vi "Launcher.vi"() -> ()   [LabVIEW 2014]
uses:
  Communication/Events/Events Lib.lvlib
  Communication/Queues/Queues Lib.lvlib
panel:
  in  "error in":errorcluster
  out "error out":errorcluster
  in  "Start Module":bool
  out "Log":string
  in  "Send Value to Chart":bool
  in  "Value":dbl
  in  "Stop Module":bool
  in  "Hide UI":bool
  in  "Show UI":bool
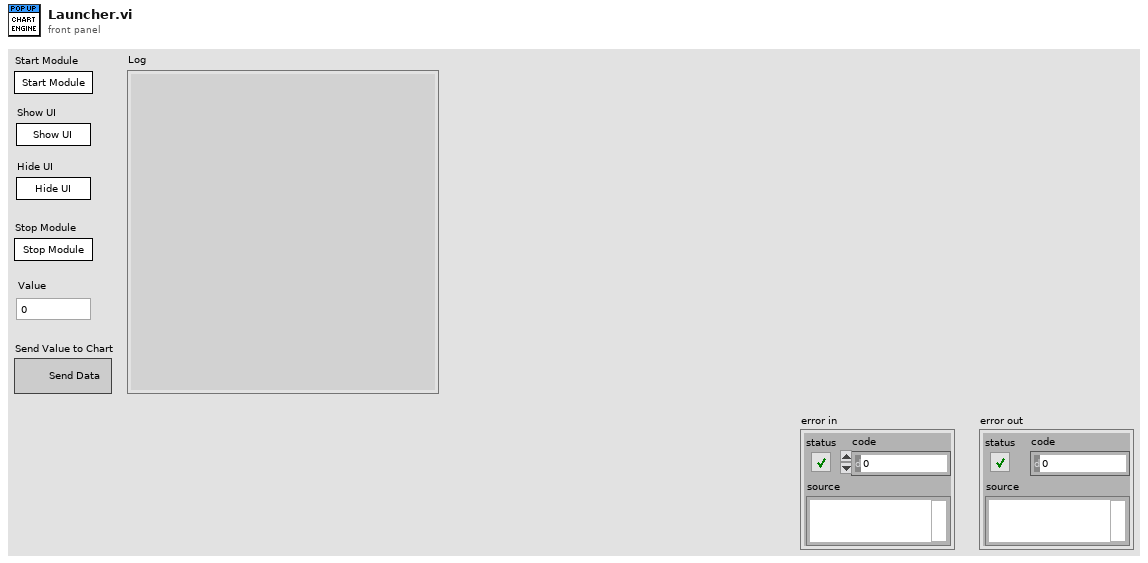
[diagram p1: front panel]
types:
  T1 = typedef "Events Lib.lvlib/Events TypeDef.ctl" = cluster{"Stop Event":refnum<user-event>, "Chart Send Value":refnum<user-event>, "Show Module":refnum<user-event>, "Hide Module":refnum<user-event>}
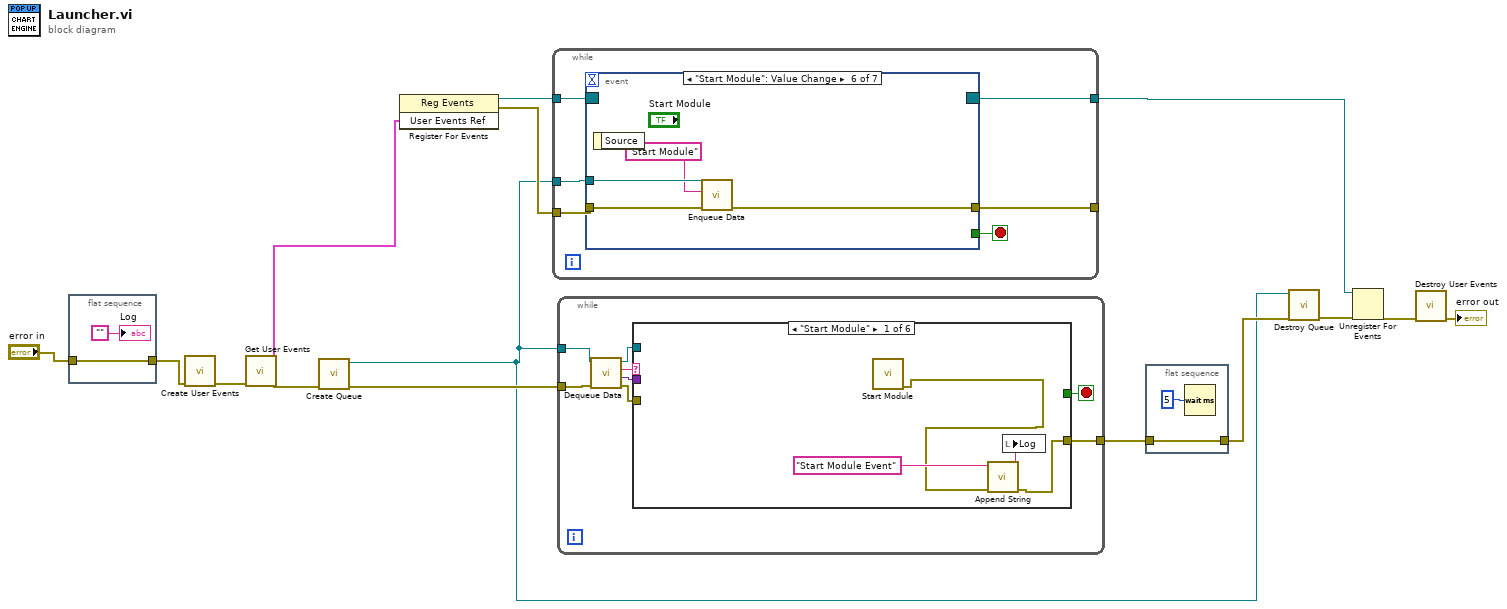
[diagram p0: block diagram]
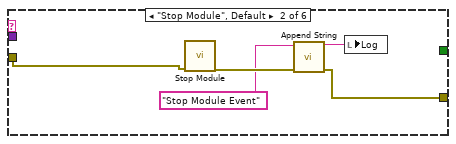
[diagram p2: hidden frame]
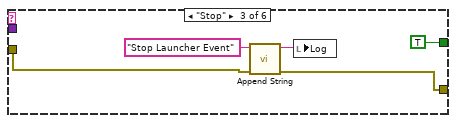
[diagram p3: hidden frame]
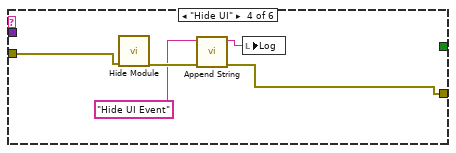
[diagram p4: hidden frame]
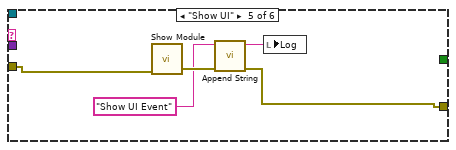
[diagram p5: hidden frame]
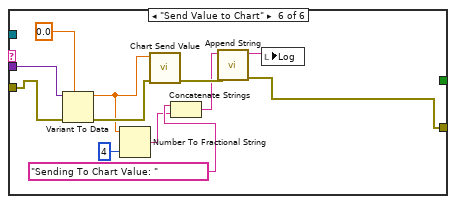
[diagram p6: hidden frame]
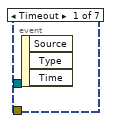
[diagram p7: hidden frame]
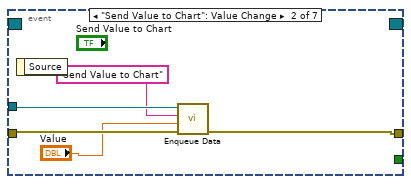
[diagram p8: hidden frame]
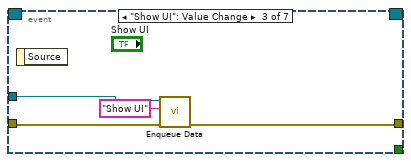
[diagram p9: hidden frame]
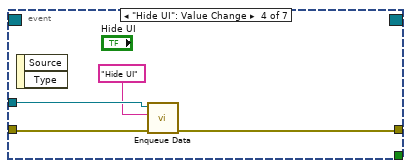
[diagram p10: hidden frame]
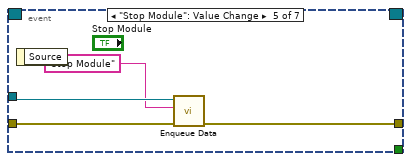
[diagram p11: hidden frame]
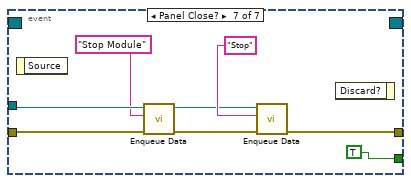
[diagram p12: hidden frame]
diagram:
  n1 = flat-sequence {
    tunnel: "error in" -> [w16]
    tunnel: [w16] -> w1
    frame #0 {
      "Log" <- ""
    }
  }
  n2 = call "Create User Events.vi"("error in"=w1) -> ("error out"=w3:errorcluster)  [unwired: 9 in, 1 out]
  n3 = call "Get User Events.vi"("error in"=w3) -> ("error out"=w13:errorcluster, "User Events Ref"=w14:T1)  [unwired: 9 in]
  n4 = call "Create Queue.vi"("error in (no error)"=w13) -> ("error out"=w12:errorcluster, "queue out"=w6:refnum<queue>)  [unwired: 9 in]
  n5 = register-events(w14) -> (reference out=w15:refnum<event-registration>, error out=w11:errorcluster)  [unwired: 2 in]
  n6 = while {
    tunnel: w15 -> [w23]
    tunnel: w6 -> [w22]
    tunnel: w11 -> [w21]
    tunnel: [w20] -> _
    tunnel: [w19] -> w10
    stop <- w18 stop-if-true
    n7 = event shown="[5] \"Start Module\": Value Change" {
      selector: w23 -> [_ _ _ _ _ _ _]
      dyn-events: [_ _ _ _ _ _ _] -> w19
      timeout: _ -> [_ _ _ _ _ _ _]
      tunnel: w22 -> [_ w28 w32 w36 w40 w44 w47]
      tunnel: w21 -> [_ w27 w31 w35 w39 w43 w46]
      tunnel: [_ w26 w29 w34 w37 w41 w52] -> w20
      tunnel: [_ _ _ _ _ _ TRUE] -> w18
      event Timeout {
        n8 = event-data() -> ()  [unwired: 1 in, 3 out]
      }
      event "Send Value to Chart": Value Change {
        n9 = event-data() -> ()  [unwired: 1 in, 1 out]
        n10 = call "Enqueue Data.vi"("error in (no error)"=w27, "Data"="Value", "Message"="Send Value to Chart", "queue in"=w28) -> ("error out"=w26:errorcluster)  [unwired: 6 in, 1 out]
      }
      event "Show UI": Value Change {
        n11 = event-data() -> ()  [unwired: 1 in, 1 out]
        n12 = call "Enqueue Data.vi"("error in (no error)"=w31, "Message"="Show UI", "queue in"=w32) -> ("error out"=w29:errorcluster)  [unwired: 7 in, 1 out]
      }
      event "Hide UI": Value Change {
        n13 = event-data() -> ()  [unwired: 1 in, 2 out]
        n14 = call "Enqueue Data.vi"("error in (no error)"=w35, "Message"="Hide UI", "queue in"=w36) -> ("error out"=w34:errorcluster)  [unwired: 7 in, 1 out]
      }
      event "Stop Module": Value Change {
        n15 = event-data() -> ()  [unwired: 1 in, 1 out]
        n16 = call "Enqueue Data.vi"("error in (no error)"=w39, "Message"="Stop Module", "queue in"=w40) -> ("error out"=w37:errorcluster)  [unwired: 7 in, 1 out]
      }
      event "Start Module": Value Change {
        n17 = event-data() -> ()  [unwired: 1 in, 1 out]
        n18 = call "Enqueue Data.vi"("error in (no error)"=w43, "Message"="Start Module", "queue in"=w44) -> ("error out"=w41:errorcluster)  [unwired: 7 in, 1 out]
      }
      event Panel Close? {
        n19 = event-data() -> ()  [unwired: 1 in, 1 out]
        n20 = call "Enqueue Data.vi"("error in (no error)"=w46, "Message"="Stop Module", "queue in"=w47) -> ("error out"=w48:errorcluster, "queue out"=w49:refnum<queue>)  [unwired: 7 in]
        n21 = call "Enqueue Data.vi"("error in (no error)"=w48, "Message"="Stop", "queue in"=w49) -> ("error out"=w52:errorcluster)  [unwired: 7 in, 1 out]
        n22 = event-data() -> ()  [unwired: 2 in, 1 out]
      }
    }
  }
  n23 = while {
    tunnel: w12 -> [w60]
    tunnel: w6 -> [w59]
    tunnel: [w54] -> w8
    stop <- w53 stop-if-true
    n24 = call "Dequeue Data.vi"("error in (no error)"=w60, "queue in"=w59) -> ("error out"=w55:errorcluster, "Data"=w56:variant, "Message"=w58:string, "queue out"=w57:refnum<queue>)  [unwired: 6 in]
    n25 = case shown="\"Start Module\"" w58 {
      tunnel: w57 -> [_ _ _ _ _ _]
      tunnel: w56 -> [_ _ _ _ _ w96]
      tunnel: w55 -> [_ w69 w72 w79 w84 w94]
      tunnel: [w62 w68 w73 w77 w82 w91] -> w54
      tunnel: [_ _ TRUE _ _ _] -> w53
      frame "Start Module" {
        n26 = call "Start Module.vi"() -> ("error out"=w61:errorcluster)  [unwired: 11 in]
        n27 = call "Append String.vi"("error in"=w61, "String to Append"="Start Module Event") -> ("error out"=w62:errorcluster, "String Out"=w63:string)  [unwired: 8 in]
        n28 = local write "Log"(w63) -> ()
      }
      frame "Stop Module", Default {
        n29 = call "Stop Module.vi"("error in"=w69) -> ("error out"=w67:errorcluster)  [unwired: 10 in]
        n30 = call "Append String.vi"("error in"=w67, "String to Append"="Stop Module Event") -> ("error out"=w68:errorcluster, "String Out"=w66:string)  [unwired: 8 in]
        n31 = local write "Log"(w66) -> ()
      }
      frame "Stop" {
        n32 = call "Append String.vi"("error in"=w72, "String to Append"="Stop Launcher Event") -> ("error out"=w73:errorcluster, "String Out"=w70:string)  [unwired: 8 in]
        n33 = local write "Log"(w70) -> ()
      }
      frame "Hide UI" {
        n34 = call "Hide Module.vi"("error in"=w79) -> ("error out"=w78:errorcluster)  [unwired: 10 in]
        n35 = call "Append String.vi"("error in"=w78, "String to Append"="Hide UI Event") -> ("error out"=w77:errorcluster, "String Out"=w76:string)  [unwired: 8 in]
        n36 = local write "Log"(w76) -> ()
      }
      frame "Show UI" {
        n37 = call "Show Module.vi"("error in"=w84) -> ("error out"=w83:errorcluster)  [unwired: 10 in]
        n38 = call "Append String.vi"("error in"=w83, "String to Append"="Show UI Event") -> ("error out"=w82:errorcluster, "String Out"=w81:string)  [unwired: 8 in]
        n39 = local write "Log"(w81) -> ()
      }
      frame "Send Value to Chart" {
        n40 = Variant To Data(error in=w94, type=0.0, Variant=w96) -> (data=w86:dbl, error out=w93:errorcluster)
        n41 = Number To Fractional String(number=w86, precision (6)=i16 4) -> (F-format string=w87:string)  [unwired: 2 in]
        n42 = call "Chart Send Value.vi"("error in"=w93, "Value"=w86) -> ("error out"=w92:errorcluster)  [unwired: 9 in]
        n43 = Concatenate Strings("Sending To Chart Value: " ("format string"), w87) -> (w89:string)
        n44 = call "Append String.vi"("error in"=w92, "String to Append"=w89) -> ("error out"=w91:errorcluster, "String Out"=w90:string)  [unwired: 8 in]
        n45 = local write "Log"(w90) -> ()
      }
    }
  }
  n46 = flat-sequence {
    tunnel: w8 -> [w97]
    tunnel: [w97] -> w7
    frame #0 {
      n47 = Wait (ms)(milliseconds to wait=u32 5) -> ()  [unwired: 1 out]
    }
  }
  n48 = call "Destroy Queue.vi"("error in (no error)"=w7, "queue in"=w6) -> ("error out"=w9:errorcluster)  [unwired: 9 in]
  n49 = Unregister For Events(event registration refnum=w10, error in=w9) -> (error out=w5:errorcluster)
  n50 = call "Destroy User Events.vi"("error in"=w5) -> ("error out"=→"error out":errorcluster)  [unwired: 9 in, 1 out]
